vi "AI_server.vi"(11 "Analog_Input.lvclass":refnum<class "Analog_Input.lvclass">) -> ()   [LabVIEW 2013, in "Analog_Input.lvclass"]
uses:
  Analog_Input.lvclass
  Experiment/states.ctl
  <vilib>/Platform/TimedLoop/XDataNode/timing_clust.ctl
  <vilib>/Platform/TimedLoop/XDataNode/nitl_modes.ctl
  <vilib>/Platform/TimedLoop/XDataNode/wakeup.ctl
  Experiment/Globals.vi
  <vilib>/platform/TimedLoop/XDataNode/XDataNode.xnode
  <vilib>/Platform/TimedLoop/XDataNode/XDNodeRunTimeDep.lvlib
panel:
  in  "error in":errorcluster
  out "Wattage chart":dbl[][](graph)
  out "watts":dbl[](array[numeric])=[8.096373353174213, 0.029310863509207197, 8.062512384255392] format="%#_4g"
  in  "scaling":dbl[](array[numeric])=[3.84, 1.48, 5.0]
  out "remote address":string
  in  "samples per channel":i32=100
  out "received message":string
  in  "shutdown":bool caption="quit"
  in  "halt":bool caption="quit"
  out "voltage":dbl[](array[numeric])=[0.013400376783720991, 0.017345916304433388]
  out "coupling chart":dbl(graph)=0.7725378439821038
  in  "descriptions":string[](array[string])
  in  "sample rate (Hz)":dbl=1000.0
  in  "physical channels":tag="PXI1Slot7/ai0:2"
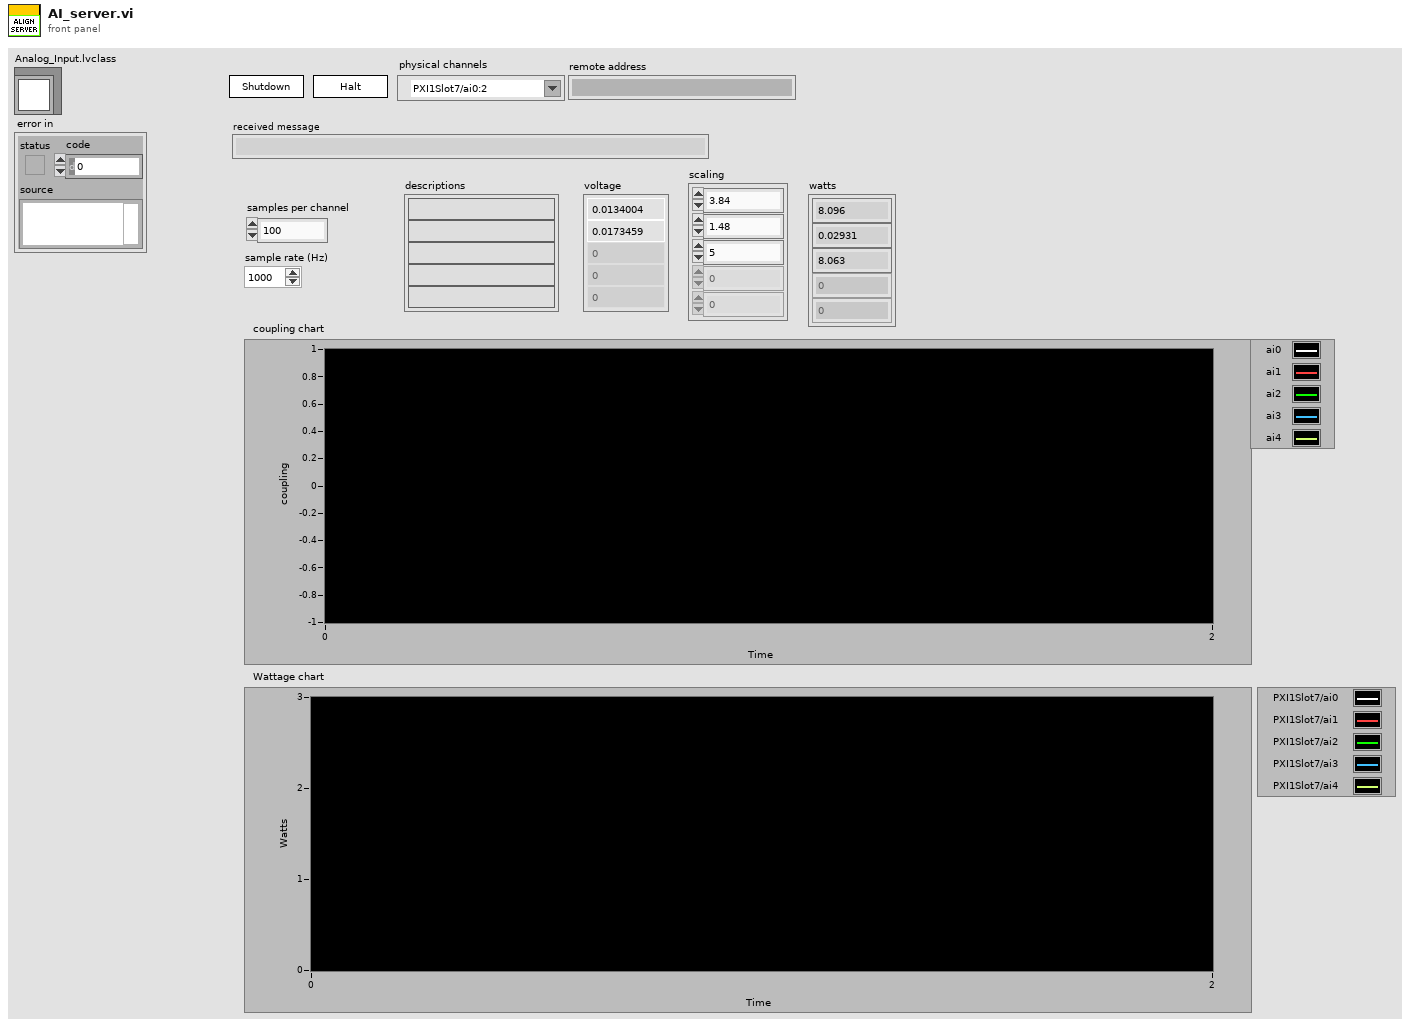
[diagram p1: front panel]
types:
  T1 = typedef "XDNodeRunTimeDep.lvlib/timing_clust.ctl" = cluster{"Expected End [f-1]":u64, "Actual End [f-1]":u64, "Finished Late? [f-1]":bool, "Expected End [i-1]":u64, "Actual End [i-1]":u64, "Finished Late? [i-1]":bool, "Expected Start [i]":u64, "Actual Start [i]":u64, "Expected Start [f]":u64, "Actual Start [f]":u64, "Source Name":string, "Structure Name":string, "Period":i64, "Deadline":i64, "Offset":i64, "Start":i64, "Priority":i32, "Timeout":i32, "Mode":T2, "Wakeup Reason":T3, "Error":errorcluster, "Source Type":string, "Secondary Source Type":string, "Global End Time":u64, "Global Start Time":u64, "Frame Duration":u64, "Iteration Duration":u64, "Assigned CPU":i32, "I/O Scan Engine Mode":u32}
  T2 = typedef "XDNodeRunTimeDep.lvlib/nitl_modes.ctl" = enum32{"No Change", "Process missed periods, maintain original phase", "Discard missed periods, maintain original phase", "Process missed periods, ignore original phase", "Discard missed periods, ignore original phase"}
  T3 = typedef "XDNodeRunTimeDep.lvlib/wakeup.ctl" = enum32{"Normal", "Aborted", "Asynchronous wakeup", "Timing source error", "Timed loop error", "Timeout"}
  T4 = typedef "states.ctl" = enum16{"run", "pause", "shutdown gracefully", "halt immediately", "waiting for connection", "waiting for command"}
  T5 = enum16{"Standard", "Buffered", "CRLF", "Immediate"}
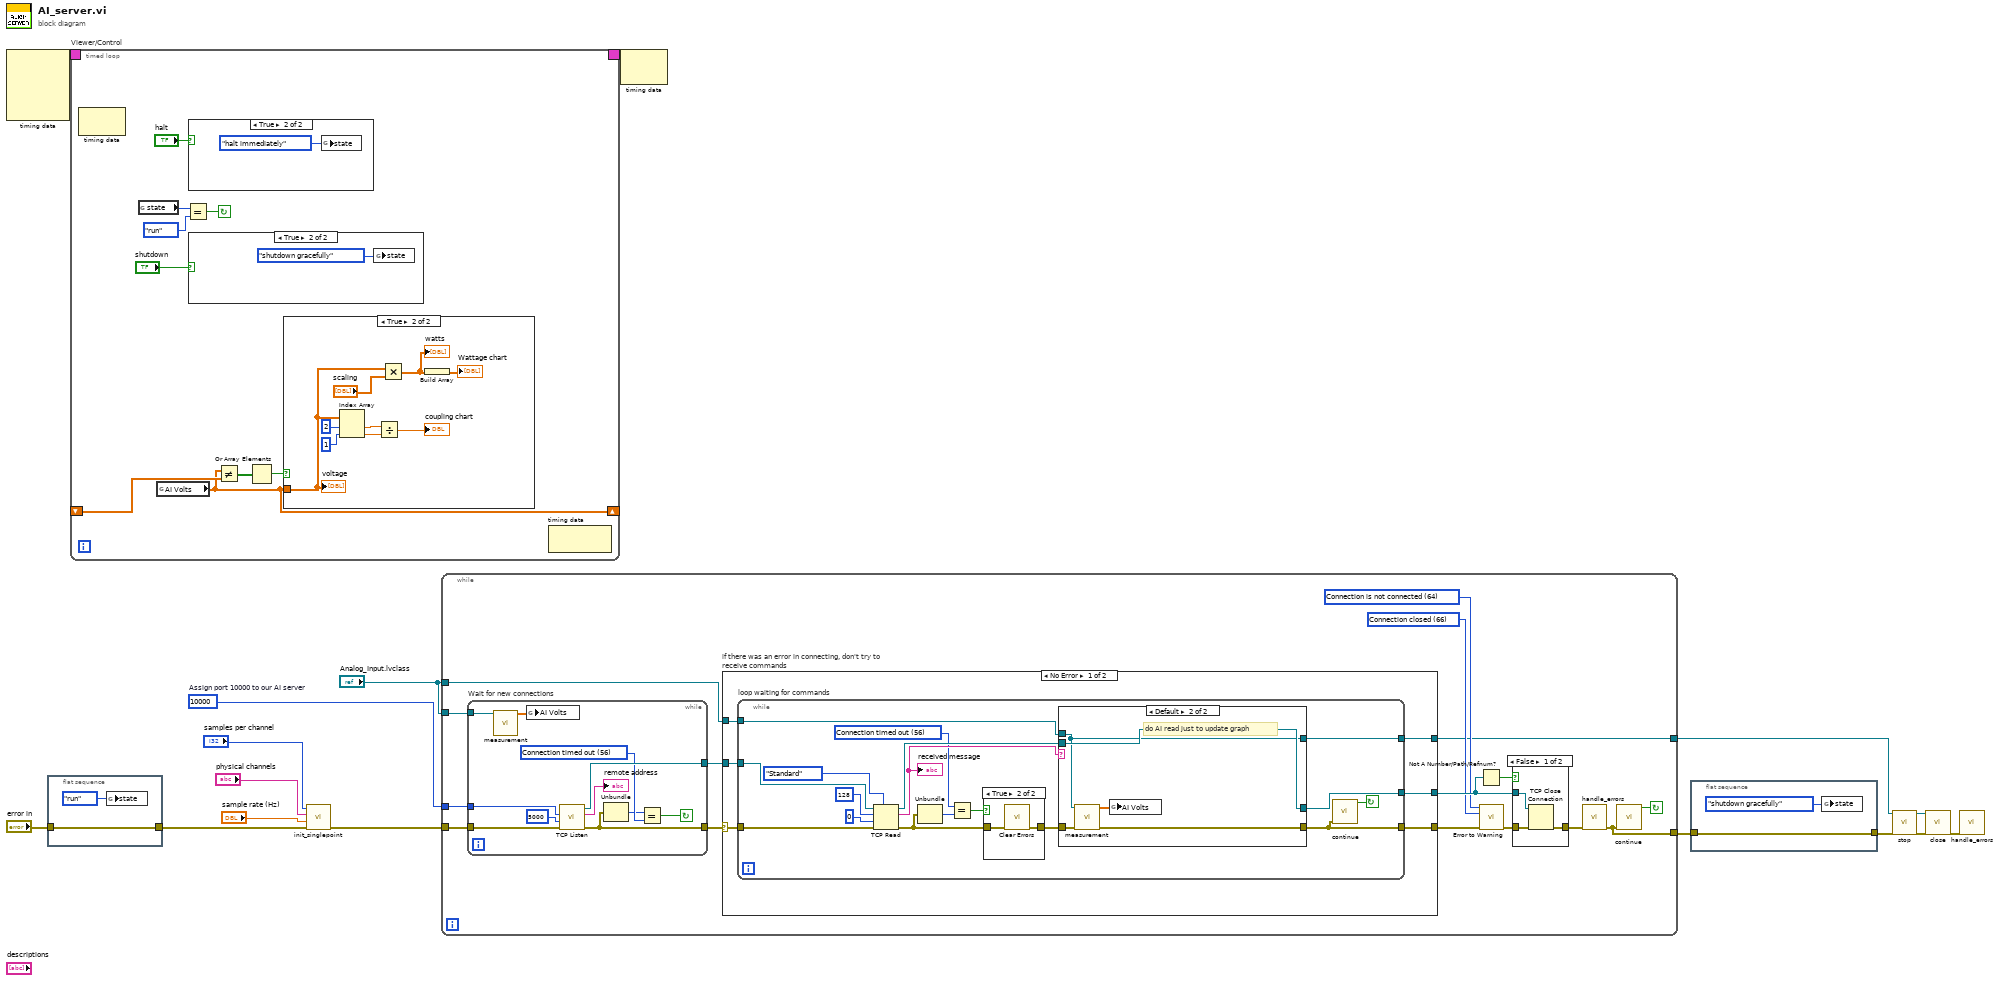
[diagram p0: block diagram]
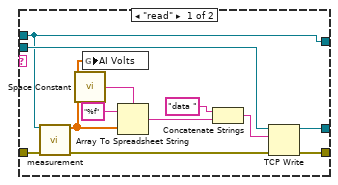
[diagram p3: hidden frame]
diagram:
  w9 = u16 10000  # Assign port 10000 to our AI server
  n1 = node-c288() -> (w16:T1)  [unwired: 4 in]
  n2 = flat-sequence {
    tunnel: [w17] -> w4
    tunnel: "error in" -> [w17]
    frame #0 {
      n3 = global write "Globals.vi" "state"(states."run" ("state")) -> ()
    }
  }
  n4 = timed-loop "Viewer/Control" {
    timing: w16 -> [_]
    timing-out: [_] -> w15
    shift-right: [w23] -> _
    shift-left: _ -> [w24]
    stop <- w25 continue-if-true
    n5 = node-c288() -> ()  [unwired: 1 in, 1 out]
    n6 = global read "Globals.vi" "state"() -> (w20:T4)
    n7 = global read "Globals.vi" "AI Volts"() -> (w23:dbl[])
    n8 = Equal?(x=w20, y=states."run" ("state")) -> (x = y?=w25:bool)
    n9 = case shown="True" "halt" {
      frame False {
      }
      frame True {
        n10 = global write "Globals.vi" "state"(states."halt immediately" ("state")) -> ()
      }
    }
    n11 = case shown="True" "shutdown" {
      frame False {
      }
      frame True {
        n12 = global write "Globals.vi" "state"(states."shutdown gracefully" ("state")) -> ()
      }
    }
    n13 = Not Equal?(x=w23, y=w24) -> (x != y?=w22:bool[])
    n14 = Or Array Elements(Boolean array=w22) -> (logical OR=w21:bool)
    n15 = case shown="True" w21 {
      tunnel: w23 -> [_ w31]
      frame False {
      }
      frame True {
        n16 = Index Array(array=w31, index #1=2 ("index"), index #2=1 ("index")) -> (element #1=w34:dbl, element #2=w33:dbl)
        n17 = Divide(x=w34, y=w33) -> (x/y=→"coupling chart":dbl)
        n18 = Multiply(x=w31, y="scaling") -> (x*y=w29:dbl[])
        "watts" <- w29
        n19 = Build Array(w29) -> (→"Wattage chart":dbl[][])
        "voltage" <- w31
      }
    }
    n20 = node-c288() -> ()  [unwired: 1 in, 1 out]
  }
  n21 = call "init_singlepoint.vi"("error in"=w4, "sample rate (Hz)"="sample rate (Hz)", "physical channels"="physical channels", "samples per channel"="samples per channel") -> ("error out"=w8:errorcluster)  [unwired: 6 in, 1 out]
  n22 = while {
    tunnel: [w44] -> w6
    tunnel: w9 -> [w56]
    tunnel: w8 -> [w48]
    tunnel: "Analog_Input.lvclass" -> [w43]
    tunnel: "Analog_Input.lvclass" -> [w42]
    tunnel: [w41] -> w1
    stop <- w47 continue-if-true
    w51 = 66 items=["No Error", "Argument Error", "Memory Full", "Out of Zone", "End of File", "File Already Open", "Generic File IO Error", "File Not Found", "File Permission Error", "Disk Full", "Duplicate Path", "Too Many Files Open", "Not Enabled", "Resource File Not Found", "Cannot Add Resource", "Resource Not Found", "Image Not Found", "Image Memory Error", "Pen Does Not Exist", "Config Bad Type", "Config Token Not Found", "Config Parse Error", "Config Memory Error", "Bad External Code Format", "Bad External Code Offset", "External Code Not Present", "Null Window", "Destroy Window Mixup", "Null Menu", "Print Aborted", "Bad Print Record", "Print Driver Error", "Windows Error During Print", "Memory Error During Print", "Print Dialog Error", "Generic Print Error", "Invalid Device Refnum", "Device Not Found", "Device Parameter Error", "Device Unit Error", "Can't Open Device", "Device Call Aborted", "Generic Error", "Cancelled By User", "Object ID Too Low", "Object ID Too High", "Object Not In Heap", "Unknown Heap", "Bad DefProc ID", "DefProc Not In Table", "Message Out Of Range", "Null Method", "Unknown Message", "Manager Call Not Supported", "Bad address", "Connection In progress", "Connection timed out", "Connection is already in progress", "Network attribute not supported", "Network error", "Address in use", "System out of memory", "Connection aborted", "Connection refused", "Connection is not connected", "Connection is already connected", "Connection closed", "Initialize error (interapplication manager)", "Bad occurrence", "Wait on unbound occurrence handler", "Occurrence queue overflow", "Bad path", "Semaphore not signaled", "Unrecognized type (interapplication manager)"] ("2nd Error to Convert")
    w52 = 64 items=["No Error", "Argument Error", "Memory Full", "Out of Zone", "End of File", "File Already Open", "Generic File IO Error", "File Not Found", "File Permission Error", "Disk Full", "Duplicate Path", "Too Many Files Open", "Not Enabled", "Resource File Not Found", "Cannot Add Resource", "Resource Not Found", "Image Not Found", "Image Memory Error", "Pen Does Not Exist", "Config Bad Type", "Config Token Not Found", "Config Parse Error", "Config Memory Error", "Bad External Code Format", "Bad External Code Offset", "External Code Not Present", "Null Window", "Destroy Window Mixup", "Null Menu", "Print Aborted", "Bad Print Record", "Print Driver Error", "Windows Error During Print", "Memory Error During Print", "Print Dialog Error", "Generic Print Error", "Invalid Device Refnum", "Device Not Found", "Device Parameter Error", "Device Unit Error", "Can't Open Device", "Device Call Aborted", "Generic Error", "Cancelled By User", "Object ID Too Low", "Object ID Too High", "Object Not In Heap", "Unknown Heap", "Bad DefProc ID", "DefProc Not In Table", "Message Out Of Range", "Null Method", "Unknown Message", "Manager Call Not Supported", "Bad address", "Connection In progress", "Connection timed out", "Connection is already in progress", "Network attribute not supported", "Network error", "Address in use", "System out of memory", "Connection aborted", "Connection refused", "Connection is not connected", "Connection is already connected", "Connection closed", "Initialize error (interapplication manager)", "Bad occurrence", "Wait on unbound occurrence handler", "Occurrence queue overflow", "Bad path", "Semaphore not signaled", "Unrecognized type (interapplication manager)"] ("1st Error to Convert")
    n23 = while "Wait for new connections" {
      tunnel: [w59] -> w46
      tunnel: [w66] -> w55
      tunnel: w56 -> [w67]
      tunnel: w48 -> [w61]
      tunnel: w42 -> [w57]
      stop <- w60 continue-if-true
      w64 = 56 items=["No Error", "Argument Error", "Memory Full", "Out of Zone", "End of File", "File Already Open", "Generic File IO Error", "File Not Found", "File Permission Error", "Disk Full", "Duplicate Path", "Too Many Files Open", "Not Enabled", "Resource File Not Found", "Cannot Add Resource", "Resource Not Found", "Image Not Found", "Image Memory Error", "Pen Does Not Exist", "Config Bad Type", "Config Token Not Found", "Config Parse Error", "Config Memory Error", "Bad External Code Format", "Bad External Code Offset", "External Code Not Present", "Null Window", "Destroy Window Mixup", "Null Menu", "Print Aborted", "Bad Print Record", "Print Driver Error", "Windows Error During Print", "Memory Error During Print", "Print Dialog Error", "Generic Print Error", "Invalid Device Refnum", "Device Not Found", "Device Parameter Error", "Device Unit Error", "Can't Open Device", "Device Call Aborted", "Generic Error", "Cancelled By User", "Object ID Too Low", "Object ID Too High", "Object Not In Heap", "Unknown Heap", "Bad DefProc ID", "DefProc Not In Table", "Message Out Of Range", "Null Method", "Unknown Message", "Manager Call Not Supported", "Bad address", "Connection In progress", "Connection timed out", "Connection is already in progress", "Network attribute not supported", "Network error", "Address in use", "System out of memory", "Connection aborted", "Connection refused", "Connection is not connected", "Connection is already connected", "Connection closed", "Initialize error (interapplication manager)", "Bad occurrence", "Wait on unbound occurrence handler", "Occurrence queue overflow", "Bad path", "Semaphore not signaled", "Unrecognized type (interapplication manager)"] ("1st Error to Convert")
      n24 = call "measurement.vi"("Analog_Input.lvclass"=w57) -> ("AI Volts"=w58:dbl[])  [unwired: 13 in, 1 out]
      n25 = global write "Globals.vi" "AI Volts"(w58) -> ()
      n26 = call <vilib>:"TCP Listen.vi"("error in (no error)"=w61, "timeout ms (wait forever: -1)"=5000, "port"=w67) -> ("error out"=w59:errorcluster, "remote address"=→"remote address":string, "connection ID"=w66:refnum<k5>)  [unwired: 4 in, 2 out]
      n27 = Unbundle(w59) -> ("code"=w63:i32)  [unwired: 2 out]
      n28 = Equal?(x=w63, y=w64) -> (x = y?=w60:bool)
    }
    n29 = case "if there was an error in connecting, don't try to receive commands" shown="No Error" w46 {
      selector: w46 -> [w70 w112]
      tunnel: [w73 w112] -> w50
      tunnel: w55 -> [w72 w113]
      tunnel: [w71 w113] -> w54
      tunnel: w43 -> [w69 w111]
      tunnel: [w68 w111] -> w41
      frame No Error {
        n30 = while "loop waiting for commands" {
          tunnel: w70 -> [w88]
          tunnel: [w83] -> w73
          tunnel: [w85] -> w71
          tunnel: w72 -> [w87]
          tunnel: w69 -> [w75]
          tunnel: [w74] -> w68
          stop <- w82 continue-if-true
          w80 = 56 items=["No Error", "Argument Error", "Memory Full", "Out of Zone", "End of File", "File Already Open", "Generic File IO Error", "File Not Found", "File Permission Error", "Disk Full", "Duplicate Path", "Too Many Files Open", "Not Enabled", "Resource File Not Found", "Cannot Add Resource", "Resource Not Found", "Image Not Found", "Image Memory Error", "Pen Does Not Exist", "Config Bad Type", "Config Token Not Found", "Config Parse Error", "Config Memory Error", "Bad External Code Format", "Bad External Code Offset", "External Code Not Present", "Null Window", "Destroy Window Mixup", "Null Menu", "Print Aborted", "Bad Print Record", "Print Driver Error", "Windows Error During Print", "Memory Error During Print", "Print Dialog Error", "Generic Print Error", "Invalid Device Refnum", "Device Not Found", "Device Parameter Error", "Device Unit Error", "Can't Open Device", "Device Call Aborted", "Generic Error", "Cancelled By User", "Object ID Too Low", "Object ID Too High", "Object Not In Heap", "Unknown Heap", "Bad DefProc ID", "DefProc Not In Table", "Message Out Of Range", "Null Method", "Unknown Message", "Manager Call Not Supported", "Bad address", "Connection In progress", "Connection timed out", "Connection is already in progress", "Network attribute not supported", "Network error", "Address in use", "System out of memory", "Connection aborted", "Connection refused", "Connection is not connected", "Connection is already connected", "Connection closed", "Initialize error (interapplication manager)", "Bad occurrence", "Wait on unbound occurrence handler", "Occurrence queue overflow", "Bad path", "Semaphore not signaled", "Unrecognized type (interapplication manager)"] ("1st Error to Convert")
          n31 = TCP Read(connection ID=w87, bytes to read=128, error in (no error)=w88, 7:T5."Standard" ("mode (standard)"), 9:0) -> (connection ID out=w86:refnum<k5>, data out=w84:string, error out=w78:errorcluster)
          "received message" <- w84
          n32 = Unbundle(w78) -> ("code"=w79:i32)  [unwired: 2 out]
          n33 = Equal?(x=w80, y=w79) -> (x = y?=w81:bool)
          n34 = case shown="True" w81 {
            tunnel: w78 -> [w91 w93]
            tunnel: [w91 w92] -> w77
            frame False {
            }
            frame True {
              n35 = call <vilib>:"Clear Errors.vi"("error in (no error)"=w93) -> ("error out"=w92:errorcluster)  [unwired: 6 in]
            }
          }
          n36 = case shown="Default" w84 {
            tunnel: w77 -> [w97 w109]
            tunnel: w86 -> [w98 w110]
            tunnel: [w105 w110] -> w85
            tunnel: [w104 w107] -> w83
            tunnel: w75 -> [w94 w106]
            tunnel: [w94 w106] -> w74
            frame "read" {
              n37 = call "measurement.vi"("Analog_Input.lvclass"=w94, "error in"=w97) -> ("AI Volts"=w96:dbl[], "error out"=w95:errorcluster)  [unwired: 12 in]
              n38 = call <vilib>:"Space Constant.vi"() -> ("String"=w102:string)
              n39 = global write "Globals.vi" "AI Volts"(w96) -> ()
              n40 = Array To Spreadsheet String(delimiter (Tab)=w102, array=w96, 3:"%f" ("format string")) -> (spreadsheet string=w101:string)
              n41 = Concatenate Strings("data " ("string"), w101) -> (w99:string)
              n42 = TCP Write(connection ID=w98, data in=w99, error in (no error)=w95) -> (connection ID out=w105:refnum<k5>, error out=w104:errorcluster)  [unwired: 1 in, 1 out]
            }
            frame Default {
              # "do AI read just to update graph"
              n43 = call "measurement.vi"("Analog_Input.lvclass"=w106, "error in"=w109) -> ("AI Volts"=w108:dbl[], "error out"=w107:errorcluster)  [unwired: 12 in]
              n44 = global write "Globals.vi" "AI Volts"(w108) -> ()
            }
          }
          n45 = call "continue.vi"("error in"=w83) -> ("continue?"=w82:bool)  [unwired: 10 in]
        }
      }
      frame Error {
      }
    }
    n46 = Not A Number/Path/Refnum?(number/path/refnum=w54) -> (NaN/Path/Refnum?=w53:bool)
    n47 = call <vilib>:"Error to Warning.vi"("1st Error to Convert"=w52, "2nd Error to Convert"=w51, "error in"=w50) -> ("warning out"=w49:errorcluster)  [unwired: 12 in]
    n48 = case shown="False" w53 {
      tunnel: w49 -> [w116 w117]
      tunnel: w54 -> [w115 _]
      tunnel: [w114 w117] -> w45
      frame False {
        n49 = TCP Close Connection(connection ID=w115, error in (no error)=w116) -> (error out=w114:errorcluster)  [unwired: 1 in, 1 out]
      }
      frame True {
      }
    }
    n50 = call "handle_errors.vi"("error in (no error)"=w45) -> ("error out"=w44:errorcluster)  [unwired: 14 in]
    n51 = call "continue.vi"("error in"=w44) -> ("continue?"=w47:bool)  [unwired: 10 in]
  }
  n52 = node-c288(w15) -> ()  [unwired: 1 out]
  n53 = flat-sequence {
    tunnel: w6 -> [w118]
    tunnel: [w118] -> w5
    frame #0 {
      n54 = global write "Globals.vi" "state"(states."shutdown gracefully" ("state")) -> ()
    }
  }
  n55 = call "stop.vi"("error in (no error)"=w5, "Analog_Input (in)"=w1) -> ("error out"=w14:errorcluster, "Analog_Input"=w2:refnum<class "Analog_Input.lvclass">)  [unwired: 8 in]
  n56 = call "close.vi"("error in (no error)"=w14, "Analog_Input (in)"=w2) -> ("error out"=w13:errorcluster)  [unwired: 8 in, 1 out]
  n57 = call "handle_errors.vi"("error in (no error)"=w13) -> ()  [unwired: 14 in, 1 out]
